vi "Edit Options.vi"(6 "Calling VI in":refnum<vi>, 8 "error in (no error)":errorcluster, 11 "Config":T1) -> (0 "error out":errorcluster, 2 "OK?":bool, 3 "Config out":T1)   [LabVIEW 2020, in "VI Properties Editor.lvlib"]
doc: "Displays a window to edit various options present in the tool."
uses:
  VI Properties Editor.lvlib
  CTLs/Config.ctl
  CTLs/Column Name.ctl
  CTLs/Filter Type.ctl
  CTLs/Filter Info.ctl
panel:
  in  "Confirm Exit?":bool caption="Confirm Exit with Unsaved Changes action"
  in  "Abbreviate Names?":bool caption="Abbreviate names"
  in  "Format Bold Tags?":bool caption="Format bold text tags"
  in  "Show Conpane Ctls Only?":bool caption="Show connector pane controls only"
  in  "Confirm Revert All?":bool caption="Confirm Revert All action"
  in  "Confirm Revert?":bool caption="Confirm Revert action"
  in  "Confirm Save All?":bool caption="Confirm Save All action"
  in  "Confirm Save?":bool caption="Confirm Save action"
  in  "Cancel":bool
  in  "OK":bool
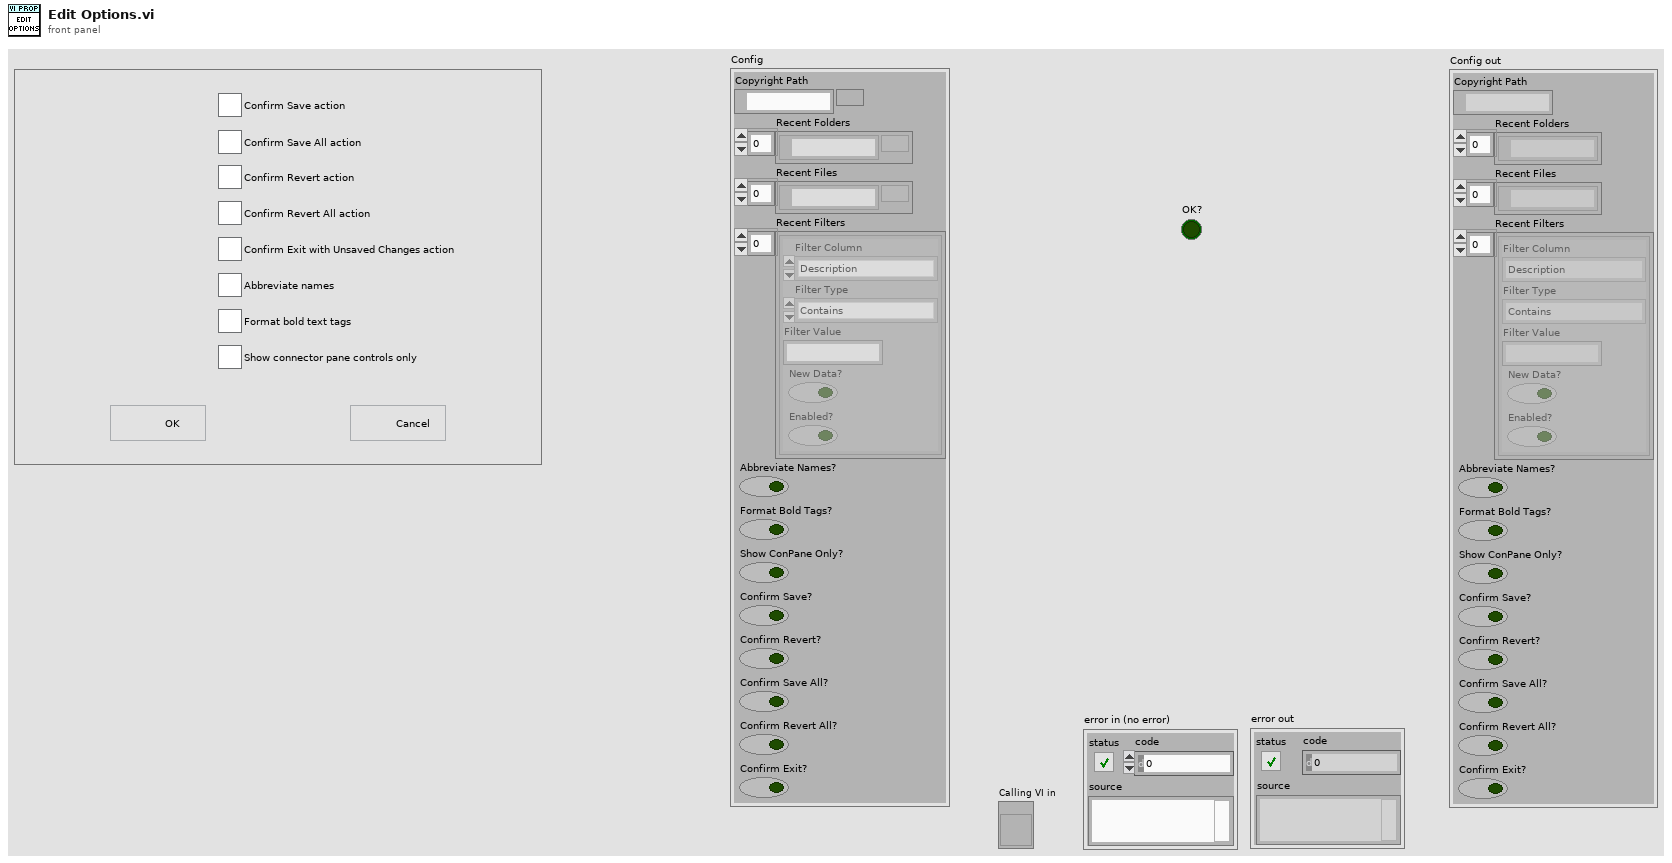
[diagram p1: front panel]
types:
  T1 = typedef "VI Properties Editor.lvlib/Config.ctl" = cluster{"Copyright Path":path, "Recent Folders":path[], "Recent Files":path[], "Recent Filters":T2[], "Abbreviate Names?":bool, "Format Bold Tags?":bool, "Show ConPane Only?":bool, "Confirm Save?":bool, "Confirm Revert?":bool, "Confirm Save All?":bool, "Confirm Revert All?":bool, "Confirm Exit?":bool}
  T2 = typedef "VI Properties Editor.lvlib/Filter Info.ctl" = cluster{"Filter Column":T3, "Filter Type":T4, "Filter Value":string, "New Data?":bool, "Enabled?":bool}
  T3 = typedef "VI Properties Editor.lvlib/Column Name.ctl" = enum16{"Name", "Path", "Type", "Window Title", "Description", "Help Path", "Help Tag", "Custom Title?", "Reentrant?", "Inlined?"}
  T4 = typedef "VI Properties Editor.lvlib/Filter Type.ctl" = enum16{"Contains", "Equals", "Starts with", "Ends with", "Does not contain", "Does not equal", "Is empty", "Is not empty"}
  T5 = enum32{"Invalid", "Standard", "Closed", "Hidden", "Minimized", "Maximized"}
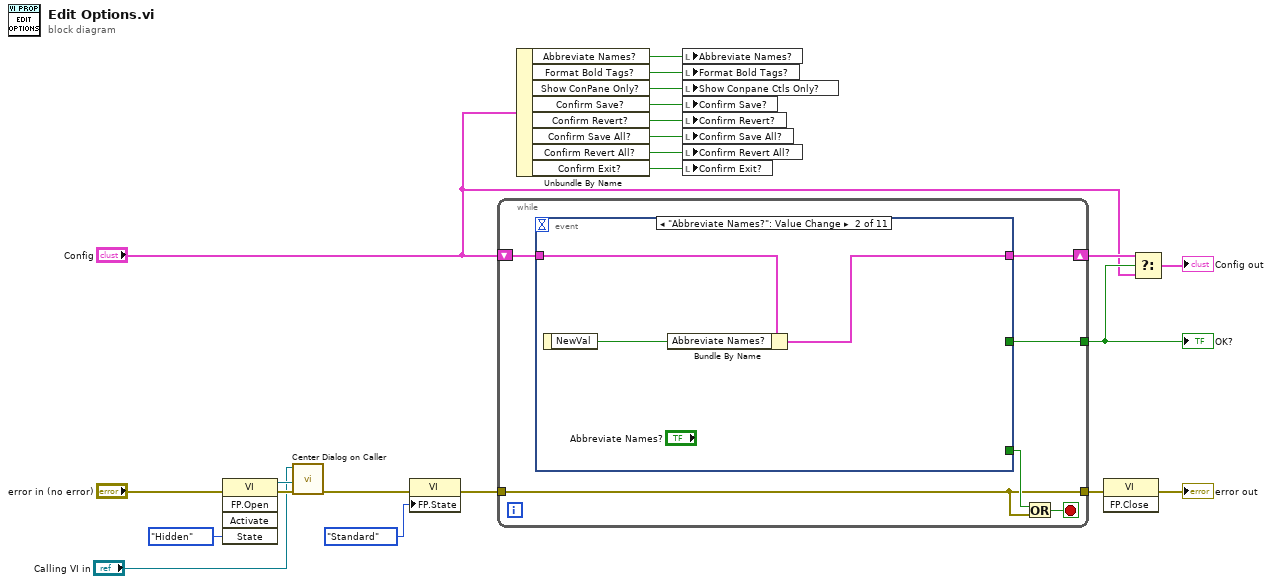
[diagram p0: block diagram]
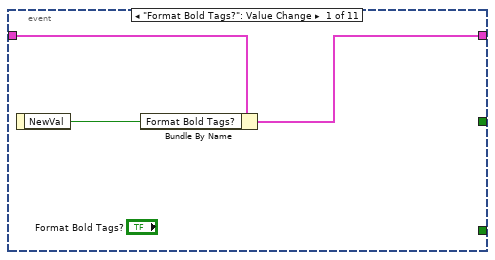
[diagram p2: hidden frame]
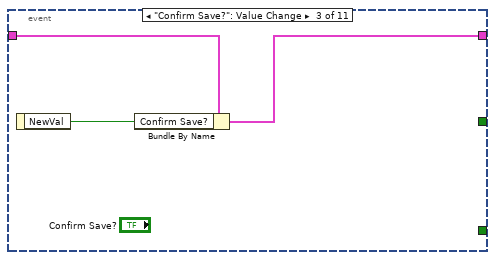
[diagram p3: hidden frame]
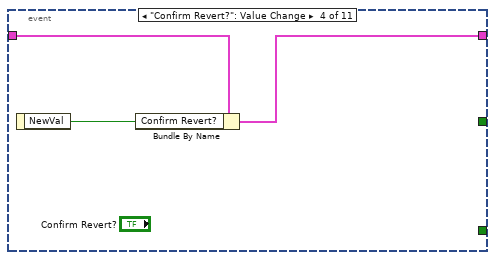
[diagram p4: hidden frame]
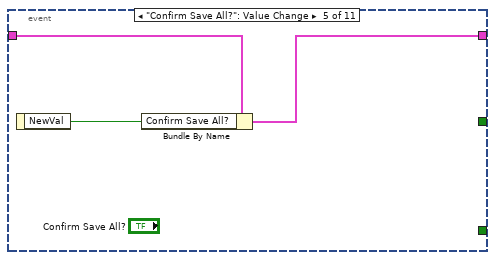
[diagram p5: hidden frame]
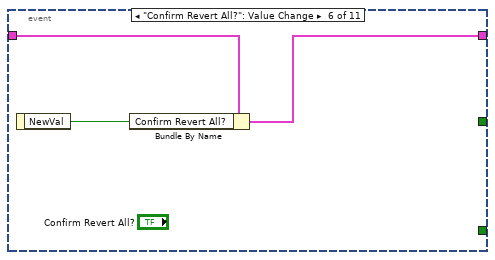
[diagram p6: hidden frame]
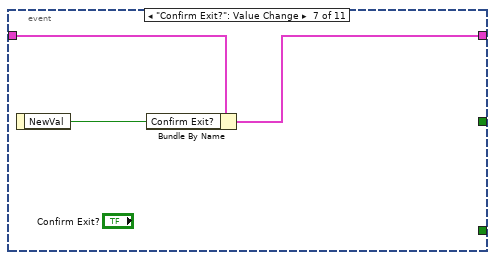
[diagram p7: hidden frame]
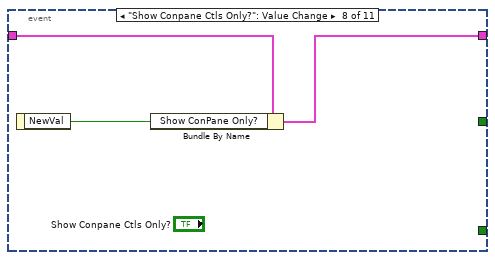
[diagram p8: hidden frame]
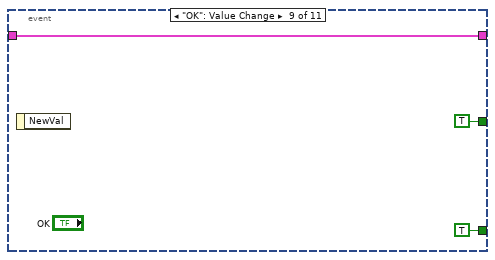
[diagram p9: hidden frame]
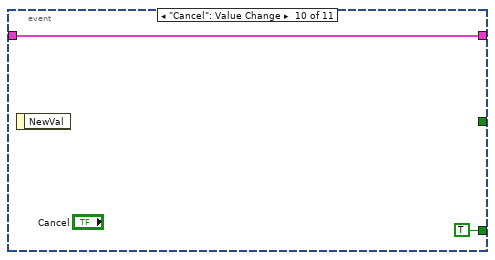
[diagram p10: hidden frame]
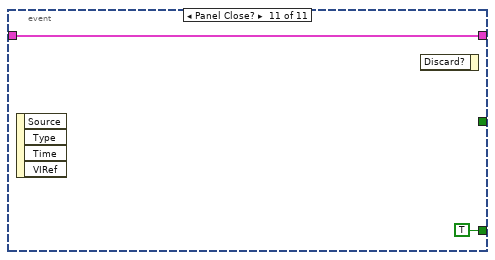
[diagram p11: hidden frame]
diagram:
  n1 = invoke class="VI" method="FP.Open"(error in="error in (no error)", "State"=T5."Hidden") -> (reference out=w7:refnum<vi>, error out=w8:errorcluster)  [unwired: 3 in, 3 out]
  n2 = call "Center Dialog on Caller.vi"("error in (no error)"=w8, "Dialog VI"=w7, "Calling VI in"="Calling VI in") -> ("error out"=w10:errorcluster)  [unwired: 7 in, 1 out]
  n3 = property class="VI"(error in=w10, "FP.State"=T5."Standard" ("Front Panel Window:State")) -> (error out=w3:errorcluster)  [unwired: 1 in, 1 out]
  n4 = while {
    shift-right: [w27] -> w15
    shift-left: "Config" -> [w28]
    tunnel: [w26] -> w14
    tunnel: w3 -> [w23]
    tunnel: [w23] -> w2
    stop <- w25 stop-if-true
    n5 = event shown="[1] \"Abbreviate Names?\": Value Change" {
      selector: _ -> [_ _ _ _ _ _ _ _ _ _ _]
      dyn-events: _ -> [_ _ _ _ _ _ _ _ _ _ _]
      timeout: _ -> [_ _ _ _ _ _ _ _ _ _ _]
      tunnel: w28 -> [w31 w34 w37 w40 w43 w46 w49 w52 w55 w57 w59]
      tunnel: [w29 w32 w35 w38 w41 w44 w47 w50 w55 w57 w59] -> w27
      tunnel: [_ _ _ _ _ _ _ _ TRUE ("NewVal") _ _] -> w26
      tunnel: [_ _ _ _ _ _ _ _ TRUE ("NewVal") TRUE ("NewVal") TRUE ("NewVal")] -> w24
      event "Format Bold Tags?": Value Change {
        n6 = event-data() -> ("NewVal"=w30:bool)  [unwired: 1 in]
        n7 = Bundle By Name(cluster=w31, "Format Bold Tags?"=w30) -> (w29:T1)
      }
      event "Abbreviate Names?": Value Change {
        n8 = event-data() -> ("NewVal"=w33:bool)  [unwired: 1 in]
        n9 = Bundle By Name(cluster=w34, "Abbreviate Names?"=w33) -> (w32:T1)
      }
      event "Confirm Save?": Value Change {
        n10 = event-data() -> ("NewVal"=w36:bool)  [unwired: 1 in]
        n11 = Bundle By Name(cluster=w37, "Confirm Save?"=w36) -> (w35:T1)
      }
      event "Confirm Revert?": Value Change {
        n12 = event-data() -> ("NewVal"=w39:bool)  [unwired: 1 in]
        n13 = Bundle By Name(cluster=w40, "Confirm Revert?"=w39) -> (w38:T1)
      }
      event "Confirm Save All?": Value Change {
        n14 = event-data() -> ("NewVal"=w42:bool)  [unwired: 1 in]
        n15 = Bundle By Name(cluster=w43, "Confirm Save All?"=w42) -> (w41:T1)
      }
      event "Confirm Revert All?": Value Change {
        n16 = event-data() -> ("NewVal"=w45:bool)  [unwired: 1 in]
        n17 = Bundle By Name(cluster=w46, "Confirm Revert All?"=w45) -> (w44:T1)
      }
      event "Confirm Exit?": Value Change {
        n18 = event-data() -> ("NewVal"=w48:bool)  [unwired: 1 in]
        n19 = Bundle By Name(cluster=w49, "Confirm Exit?"=w48) -> (w47:T1)
      }
      event "Show Conpane Ctls Only?": Value Change {
        n20 = event-data() -> ("NewVal"=w51:bool)  [unwired: 1 in]
        n21 = Bundle By Name(cluster=w52, "Show ConPane Only?"=w51) -> (w50:T1)
      }
      event "OK": Value Change {
        n22 = event-data() -> ()  [unwired: 1 in, 1 out]
      }
      event "Cancel": Value Change {
        n23 = event-data() -> ()  [unwired: 1 in, 1 out]
      }
      event Panel Close? {
        n24 = event-data() -> ()  [unwired: 1 in, 4 out]
        n25 = event-data() -> ()  [unwired: 2 in, 1 out]
      }
    }
    n26 = Or(x=w24, y=w23) -> (x .or. y?=w25:bool)
  }
  "OK?" <- w14
  n27 = Unbundle By Name("Config") -> ("Abbreviate Names?"=w16:bool, "Format Bold Tags?"=w22:bool, "Show ConPane Only?"=w21:bool, "Confirm Save?"=w20:bool, "Confirm Revert?"=w19:bool, "Confirm Save All?"=w18:bool, "Confirm Revert All?"=w17:bool, "Confirm Exit?"=w11:bool)
  n28 = local write "Abbreviate Names?"(w16) -> ()
  n29 = local write "Format Bold Tags?"(w22) -> ()
  n30 = local write "Show Conpane Ctls Only?"(w21) -> ()
  n31 = local write "Confirm Save?"(w20) -> ()
  n32 = local write "Confirm Revert?"(w19) -> ()
  n33 = local write "Confirm Save All?"(w18) -> ()
  n34 = local write "Confirm Revert All?"(w17) -> ()
  n35 = local write "Confirm Exit?"(w11) -> ()
  n36 = invoke class="VI" method="FP.Close"(error in=w2) -> (error out=→"error out":errorcluster)  [unwired: 2 in, 2 out]
  n37 = Select(t=w15, s=w14, f="Config") -> (s? t:f=→"Config out":T1)
